vi "脉冲生成(缓存)_基于频率.vi"() -> ()   [LabVIEW 2013]
uses:
  <userlib>/ArtDAQ/_SubVI/ArtDAQ_CreateCOPulseChanFreq.vi
  <userlib>/ArtDAQ/_SubVI/ArtDAQ_Write Counter Freq NSamp.vi
  <userlib>/ArtDAQ/_SubVI/ArtDAQ_CfgImplicitTiming.vi
  <userlib>/ArtDAQ/_SubVI/ArtDAQ_CfgSampClkTiming.vi
panel:
  in  "定时":enum32{"隐式时钟", "外时钟"}(tab)
  in  "时钟源":string="/Dev1/PFI0"
  in  "采样速率":dbl=1000.0
  in  "数据":cluster{"频率":dbl, "占空比":dbl}[](array[cluster])=[{"频率"=100.0, "占空比"=0.5}, {"频率"=50.0, "占空比"=0.3}, {"频率"=200.0, "占空比"=0.8}, {"频率"=100.0, "占空比"=0.5}, {"频率"=100.0, "占空比"=0.5}]
  in  "每通道采样点数":i32=4
  in  "Stop":bool
  in  "计数器":string="Dev1/ctr0"
  out "错误输出":errorcluster
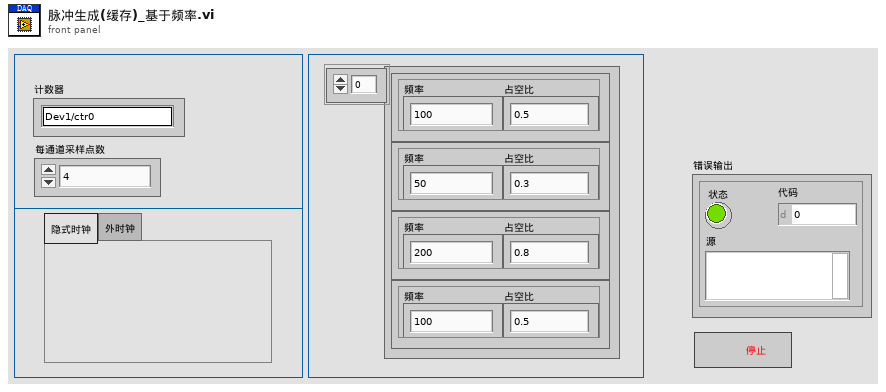
[diagram p1: front panel]
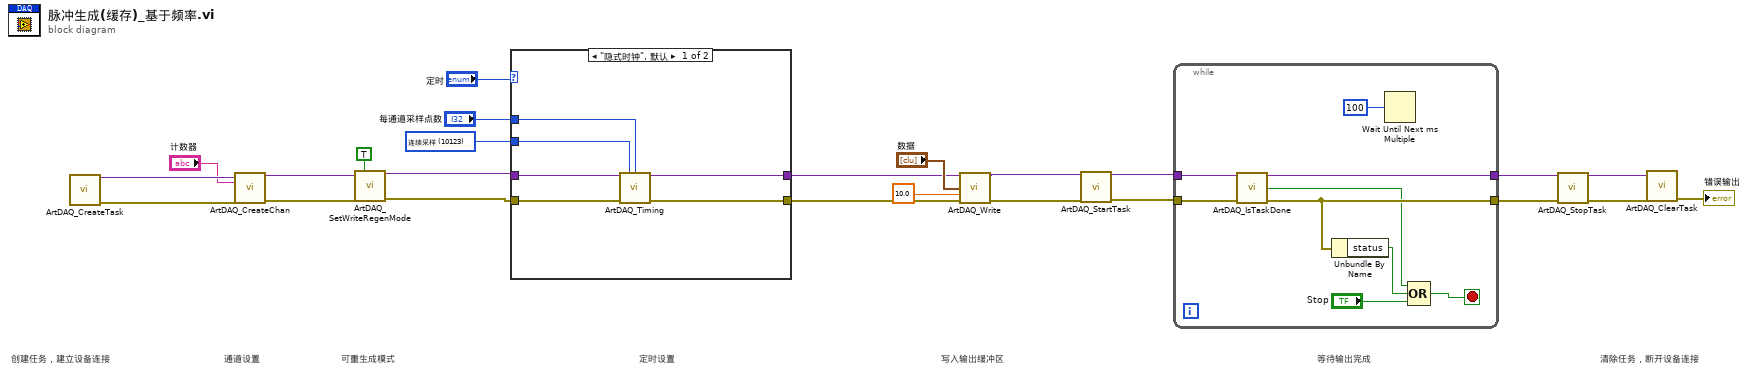
[diagram p0: block diagram]
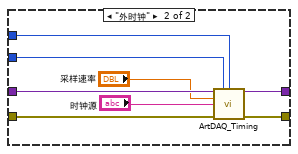
[diagram p2: hidden frame]
diagram:
  w16 = 10123 items=["有限点采样"=10178, "连续采样"=10123] ("采样模式")
  # "清除任务，断开设备连接"
  # "等待输出完成"
  # "写入输出缓冲区"
  # "定时设置"
  # "可重生成模式"
  # "通道设置"
  # "创建任务，建立设备连接"
  n1 = call <userlib>:"ArtDAQ_CreateTask.vi"() -> ("任务句柄"=w24:variant, "错误输出"=w23:errorcluster)  [unwired: 14 in]
  n2 = call-poly <userlib>:"ArtDAQ_CreateChan.vi"("任务句柄"=w24, "计数器"="计数器", "错误输入"=w23) -> ("任务句柄"=w3:variant, "错误输出"=w5:errorcluster)  [unwired: 11 in]
  n3 = call "ArtDAQ_SetWriteRegenMode.vi"("任务句柄"=w3, "可重生成？"=TRUE, "错误输入"=w5) -> ("任务句柄"=w2:variant, "错误输出"=w4:errorcluster)  [unwired: 11 in]
  n4 = case shown="\"隐式时钟\", 默认" "定时" {
    tunnel: w2 -> [w30 w38]
    tunnel: w4 -> [w29 w35]
    tunnel: w16 -> [w28 w34]
    tunnel: [w27 w37] -> w7
    tunnel: [w26 w36] -> w6
    tunnel: "每通道采样点数" -> [w25 w33]
    frame "隐式时钟", Default {
      n5 = call-poly <userlib>:"ArtDAQ_Timing.vi"("任务句柄"=w30, "采样模式"=w28, "每通道采样数"=w25, "错误输入"=w29) -> ("任务句柄"=w27:variant, "错误输出"=w26:errorcluster)  [unwired: 10 in]
    }
    frame "外时钟" {
      n6 = call-poly <userlib>:"ArtDAQ_Timing.vi"("任务句柄"=w38, "采样模式"=w34, "每通道采样数"=w33, "采样率"="采样速率", "源"="时钟源", "错误输入"=w35) -> ("任务句柄"=w37:variant, "错误输出"=w36:errorcluster)  [unwired: 8 in]
    }
  }
  n7 = call-poly <userlib>:"ArtDAQ_Write.vi"("任务句柄"=w7, "数据"="数据", "超时s"=10.0 ("Timeout"), "错误输入"=w6) -> ("任务句柄"=w8:variant, "错误输出"=w9:errorcluster)  [unwired: 9 in, 1 out]
  n8 = call <userlib>:"ArtDAQ_StartTask.vi"("任务句柄"=w8, "错误输入"=w9) -> ("任务句柄"=w15:variant, "错误输出"=w14:errorcluster)  [unwired: 12 in]
  n9 = while {
    tunnel: [w47] -> w21
    tunnel: [w46] -> w19
    tunnel: w15 -> [w43]
    tunnel: w14 -> [w42]
    stop <- w41 stop-if-true
    n10 = call <userlib>:"ArtDAQ_IsTaskDone.vi"("任务句柄"=w43, "错误输入"=w42) -> ("任务句柄"=w47:variant, "完成任务？"=w39:bool, "错误输出"=w46:errorcluster)  [unwired: 11 in]
    n11 = Unbundle By Name(w46) -> ("status"=w45:bool)
    n12 = Wait Until Next ms Multiple(millisecond multiple=u32 100 ("毫秒倍数")) -> ()  [unwired: 1 out]
    n13 = Compound Arithmetic op=OR(w39, w45, "Stop") -> (w41:bool)
  }
  n14 = call <userlib>:"ArtDAQ_StopTask.vi"("任务句柄"=w21, "错误输入"=w19) -> ("任务句柄"=w20:variant, "错误输出"=w18:errorcluster)  [unwired: 12 in]
  n15 = call <userlib>:"ArtDAQ_ClearTask.vi"("任务句柄"=w20, "错误输入"=w18) -> ("错误输出"=→"错误输出":errorcluster)  [unwired: 13 in]
